vi "FileWriteTestWindows.vi"() -> ()   [LabVIEW 2017]
uses:
  State.ctl
panel:
  in  "Next":bool
  in  "base path":path
  in  "Log File Path":path
  in  "Files Written Per Iteration":i64
  out "Elapsed Time This Iteration (ms)":u32
  out "error out":errorcluster
  in  "Folder Name in Home Directory":string
  in  "stop":bool
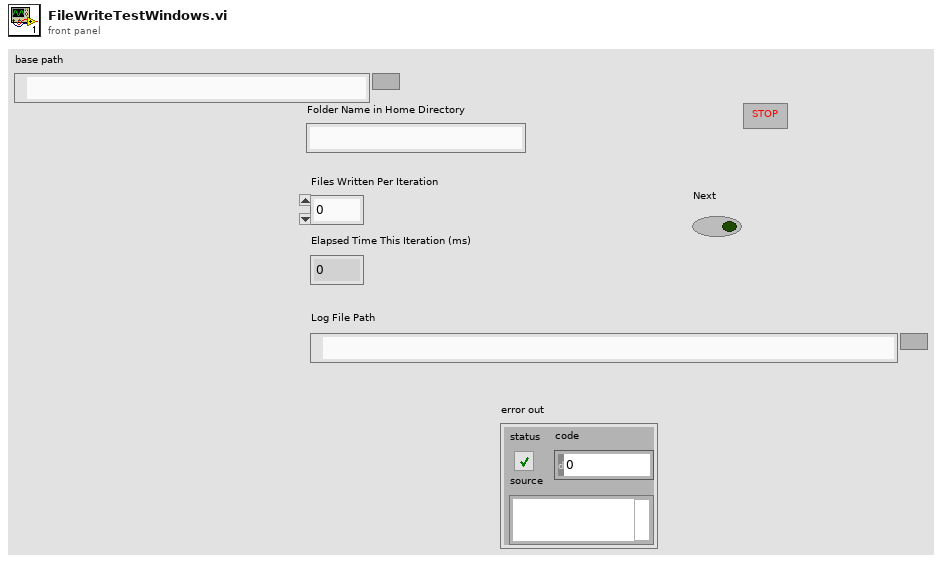
[diagram p1: front panel]
types:
  T1 = typedef "State.ctl" = enum16{"Initialize", "Write", "Log", "Stop"}
  T2 = enum16{"open", "replace", "create", "open or create", "replace or create", "replace or create with confirmation"}
  T3 = enum16{"open", "open or create", "create or replace", "create", "open (read-only)"}
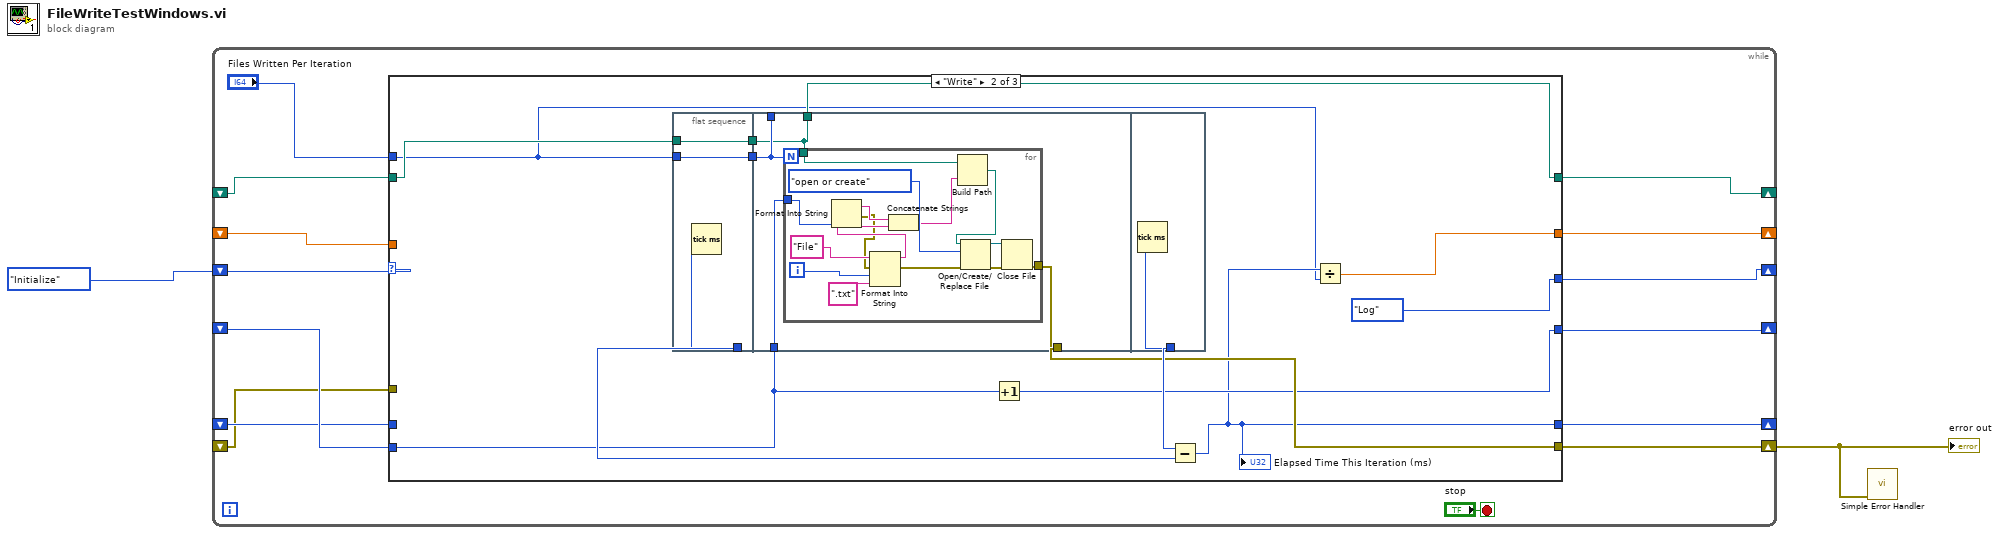
[diagram p0: block diagram]
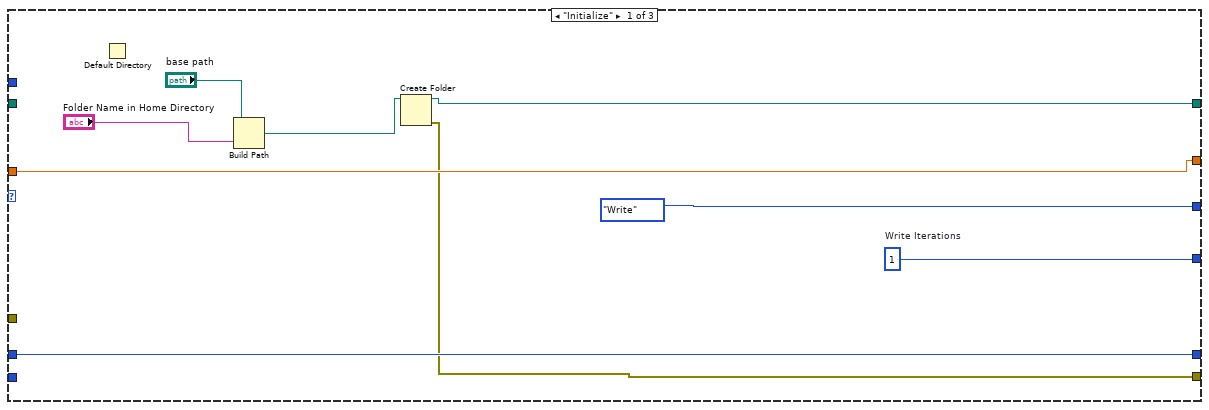
[diagram p2: hidden frame]
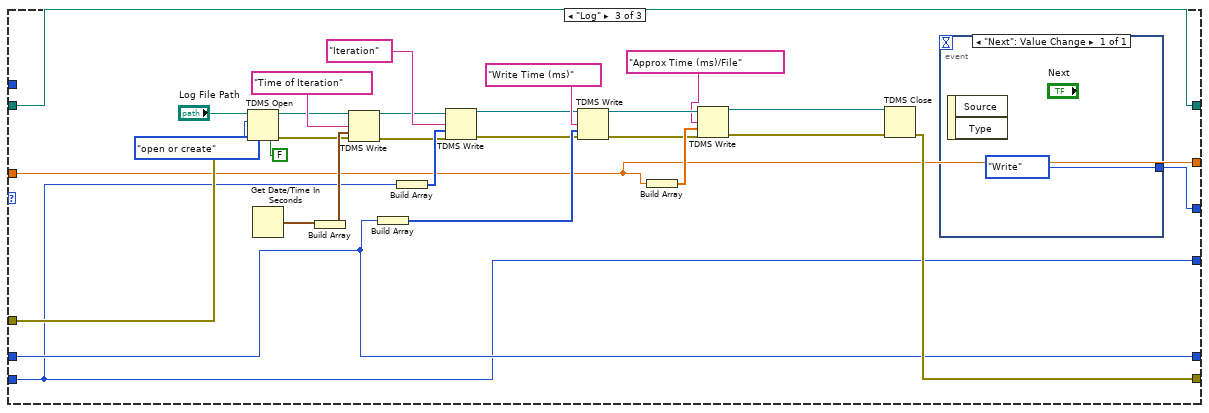
[diagram p3: hidden frame]
diagram:
  n1 = while {
    shift-right: [w3] -> _
    shift-left: State."Initialize" -> [w16]
    shift-right: [w13] -> _
    shift-left: _ -> [w12]
    shift-right: [w11] -> _
    shift-left: _ -> [w7]
    shift-right: [w10] -> w1
    shift-left: _ -> [w4]
    shift-right: [w9] -> _
    shift-left: _ -> [w8]
    shift-right: [w6] -> _
    shift-left: _ -> [w5]
    stop <- "stop" stop-if-true
    n2 = case shown="\"Write\"" w16 {
      tunnel: "Files Written Per Iteration" -> [_ w26 _]
      tunnel: [w18 w29 w63] -> w13
      tunnel: w12 -> [_ w31 w63]
      tunnel: [w22 w27 w66] -> w11
      tunnel: [w19 w35 w68] -> w10
      tunnel: [w24 w34 w65] -> w9
      tunnel: w8 -> [_ w28 w65]
      tunnel: w7 -> [w22 _ w66]
      tunnel: [w23 w33 w67] -> w6
      tunnel: w5 -> [w23 _ w67]
      tunnel: w4 -> [_ _ w74]
      tunnel: [State."Write" State."Log" w62] -> w3
      frame "Initialize" {
        w24 = 1  # Write Iterations
        n3 = Default Directory() -> ()  [unwired: 1 out]
        n4 = Build Path(base path="base path", name or relative path="Folder Name in Home Directory") -> (appended path=w20:path)
        n5 = Create Folder(path (use dialog)=w20) -> (created path=w18:path, error out=w19:errorcluster)  [unwired: 2 in, 1 out]
      }
      frame "Write" {
        n6 = flat-sequence {
          tunnel: w26 -> [w41]
          tunnel: [w41] -> w38
          tunnel: [w40] -> w36
          tunnel: w31 -> [w39]
          tunnel: [w39] -> w30
          tunnel: w38 -> [w44]
          tunnel: [w45] -> w35
          tunnel: [w44] -> _
          tunnel: w30 -> [w43]
          tunnel: [w43] -> w29
          tunnel: w28 -> [w42]
          tunnel: [w61] -> w37
          frame #0 {
            n7 = Tick Count (ms)() -> (millisecond timer value=w40:u32)
          }
          frame #1 {
            n8 = for {
              N: w44 -> [_]
              tunnel: [w53] -> w45
              tunnel: w43 -> [w52]
              tunnel: w42 -> [w48]
              i -> [w59]
              n9 = Format Into String(w48) -> (resulting string=w47:string, error out=w46:errorcluster)  [unwired: 3 in]
              n10 = Format Into String(initial string="File", error in=w46, w59, ".txt") -> (resulting string=w50:string, error out=w57:errorcluster)  [unwired: 1 in]
              n11 = Concatenate Strings(w47, w50) -> (w51:string)
              n12 = Build Path(base path=w52, name or relative path=w51) -> (appended path=w56:path)
              n13 = Open/Create/Replace File(file path (use dialog)=w56, error in=w57, operation (0:open)=T2."open or create") -> (refnum out=w55:refnum<file>, error out=w54:errorcluster)  [unwired: 3 in, 1 out]
              n14 = Close File(refnum=w55, error in=w54) -> (error out=w53:errorcluster)  [unwired: 1 out]
            }
          }
          frame #2 {
            n15 = Tick Count (ms)() -> (millisecond timer value=w61:u32)
          }
        }
        n16 = Increment(x=w28) -> (x+1=w34:i32)
        n17 = Subtract(x=w37, y=w36) -> (x-y=w27:u32)
        "Elapsed Time This Iteration (ms)" <- w27
        n18 = Divide(x=w27, y=w26) -> (x/y=w33:dbl)
      }
      frame "Log" {
        n19 = TDMS Open(6:FALSE ("disable buffering (T)"), 8:w74, 10:T3."open or create" ("operation"), 11:"Log File Path") -> (0:w73:errorcluster, 3:w87:refnum<k34>)  [unwired: 3 in]
        n20 = Get Date/Time In Seconds() -> (seconds since 1Jan1904=w86:timestamp)
        n21 = Build Array(w86) -> (w85:timestamp[])
        n22 = TDMS Write(0:w87, 7:"Time of Iteration", 9:w85, 11:w73) -> (4:w80:refnum<k34>, 15:w72:errorcluster)  [unwired: 2 in, 2 out]
        n23 = Build Array(w66) -> (w83:u32[])
        n24 = Build Array(w65) -> (w81:i32[])
        n25 = TDMS Write(0:w80, 7:"Iteration", 9:w81, 11:w72) -> (4:w79:refnum<k34>, 15:w71:errorcluster)  [unwired: 2 in, 2 out]
        n26 = TDMS Write(0:w79, 7:"Write Time (ms)", 9:w83, 11:w71) -> (4:w78:refnum<k34>, 15:w70:errorcluster)  [unwired: 2 in, 2 out]
        n27 = Build Array(w67) -> (w77:dbl[])
        n28 = TDMS Write(0:w78, 7:"Approx Time (ms)/File", 9:w77, 11:w70) -> (4:w75:refnum<k34>, 15:w69:errorcluster)  [unwired: 2 in, 2 out]
        n29 = TDMS Close(8:w69, 11:w75) -> (0:w68:errorcluster)  [unwired: 1 out]
        n30 = event shown="[0] \"Next\": Value Change" {
          selector: _ -> [_]
          dyn-events: _ -> [_]
          timeout: _ -> [_]
          tunnel: [State."Write"] -> w62
          event "Next": Value Change {
            n31 = event-data() -> ()  [unwired: 1 in, 2 out]
          }
        }
      }
    }
  }
  "error out" <- w1
  n32 = call <vilib>:"Simple Error Handler.vi"("error in (no error)"=w1) -> ()  [unwired: 4 in, 5 out]
